vi "GT Helix YZRX.vi"(0 "cardNum":i16, 1 "z":i32, 2 "circleDir":i16, 3 "synAcc":dbl, 5 "crd":i16, 7 "x":i32, 9 "y":i32, 10 "fifo":i16, 11 "error in (no error)":errorcluster caption="错误输入（无错误）", 12 "radius":dbl, 13 "synVel":dbl, 14 "velEnd":dbl) -> (4 "function return":i16, 15 "error out":errorcluster caption="错误输出")   [LabVIEW 2014, in "gts.lvlib"]
doc: "GT_API GT_HelixYZRX(short cardNum,short crd,long x,long y,long z,double radius,short circleDir,double synVel,double synAcc,double velEnd=0,short fifo=0);"
uses:
  gts.lvlib
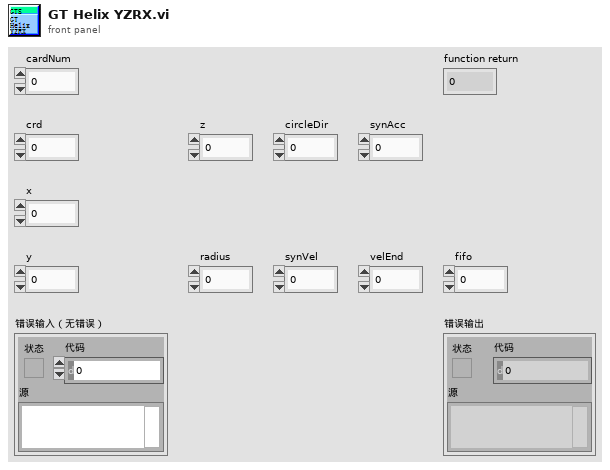
[diagram p1: front panel]
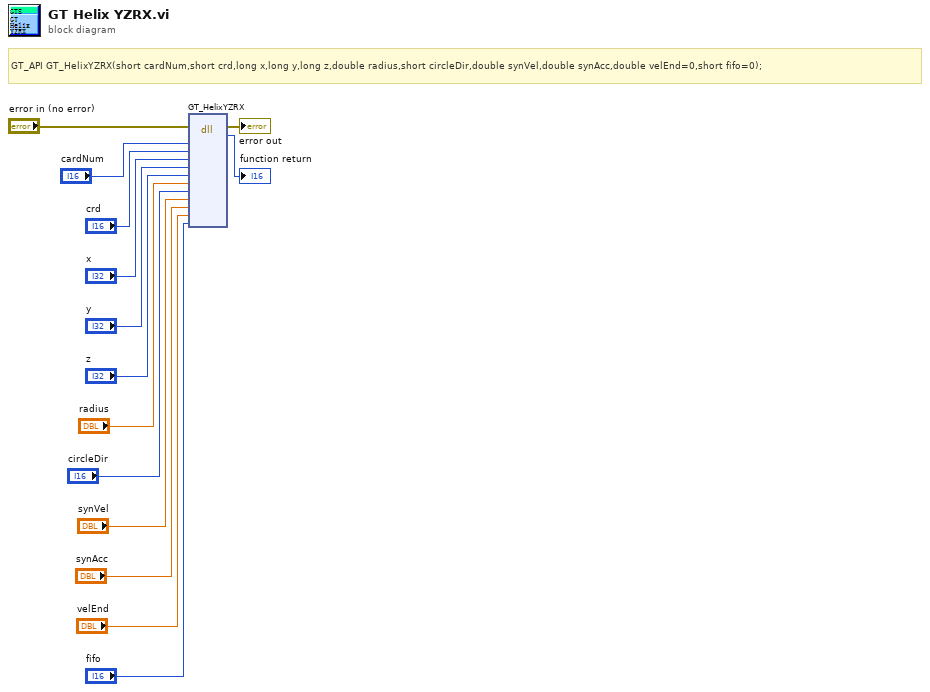
[diagram p0: block diagram]
diagram:
  # "GT_API GT_HelixYZRX(short cardNum,short crd,long x,long y,long z,double radius,short circleDir,double synVel,double synAcc,double velEnd=0,short fifo=0);"
  n1 = dll-call lib="PTH2habs D固高科技资料GTS控制卡GTS卡18年上半年资料dllVC32bit\nmulti_cardgts.*" fn="GT_HelixYZRX"(error in="error in (no error)", "cardNum"="cardNum", "crd"="crd", "x"="x", "y"="y", "z"="z", "radius"="radius", "circleDir"="circleDir", "synVel"="synVel", "synAcc"="synAcc", "velEnd"="velEnd", "fifo"="fifo") -> (error out=→"error out":errorcluster, →"function return":i16)  [unwired: 13 in, 1 out]
